vi "ResetTrackingParameters.vi"(8 "tracking parameters in":T1, 11 "Manual Threshold":cluster{sgl, sgl}(slide)={195.99734, 255.0} caption="Threshold Range" scale=0.0..255.0) -> (0 "tracking parameters out":T1)   [LabVIEW 2013]
uses:
  TrackingParameters.ctl
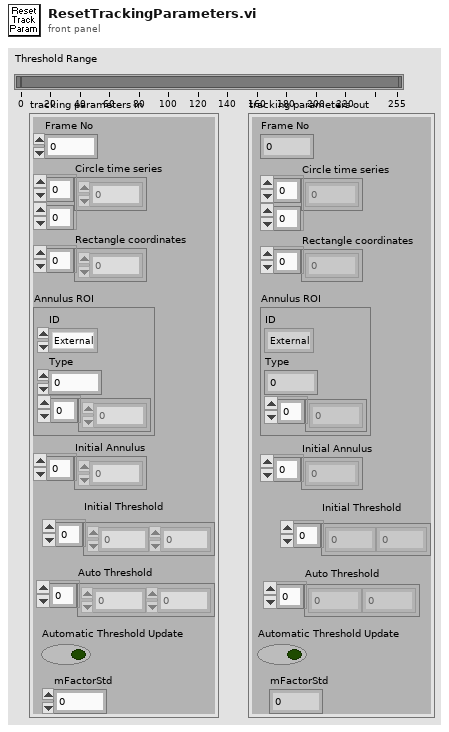
[diagram p1: front panel]
types:
  T1 = typedef "TrackingParameters.ctl" = cluster{"Frame No":i32, "Circle time series":dbl[][], "Rectangle coordinates":i32[], "Annulus ROI":cluster{"ID":enum32{"External", "Internal"}, "Type":u32, i32[]}, "Initial Annulus":i32[], "Auto Threshold":sgl[], "Automatic Threshold Update":bool, "Initial Threshold":sgl[], "mFactorStd":dbl}
  T2 = cluster{"ID":enum32{"External", "Internal"}, "Type":u32, "Initial Annulus":i32[]}
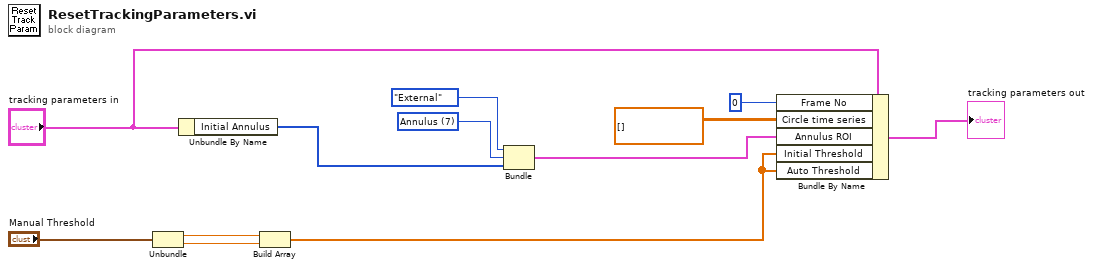
[diagram p0: block diagram]
diagram:
  w7 = u32 7 items=["No Selection", "Point", "Line", "Rectangle", "Oval", "Polygon", "Freehand Region", "Annulus", "Unused2", "Unused3", "Broken Line", "Freehand Line", "Rotated Rectangle"] ("Type")
  n1 = Unbundle("Manual Threshold") -> (w3:sgl, w2:sgl)
  n2 = Unbundle By Name("tracking parameters in") -> ("Initial Annulus"=w6:i32[])
  n3 = Build Array(w3, w2) -> (w1:sgl[])
  n4 = Bundle("ID"=enum32{"External", "Internal"}."External", "Type"=w7, "Initial Annulus"=w6) -> (w5:T2)  [unwired: 1 in]
  n5 = Bundle By Name(cluster="tracking parameters in", "Frame No"=0, "Circle time series"=dbl[][] [], "Annulus ROI"=w5, "Initial Threshold"=w1, "Auto Threshold"=w1) -> (→"tracking parameters out":T1)
